vi "Find Yellow.vi"(6 "error in":errorcluster, 9 "SS File Path":path=path "C:/PokerSS/SS.png") -> (0 "error out":errorcluster, 3 "Yellow Player":dbl)   [LabVIEW 2015]
uses:
  <vilib>/vision/NI_Vision_Development_Module.lvlib
panel:
  in  "Grid for Yellow Player":dbl[][](array[numeric])=[[1041.0, 471.0, 1195.0, 510.0], [1226.0, 513.0, 1379.0, 553.0], [1368.0, 674.0, 1521.0, 715.0], [1235.0, 807.0, 1393.0, 856.0], [1004.0, 835.0, 1161.0, 885.0], [735.0, 844.0, 893.0, 885.0], [518.0, 810.0, 680.0, 854.0], [363.0, 668.0, 522.0, 709.0], [505.0, 510.0, 662.0, 554.0], [697.0, 475.0, 855.0, 514.0]]
  out "Found Yellow":bool
  in  "Minimum Match Score (Find Yellow)":sgl=800.0
  in  "Number of Matches Requested (Find Yellow)":i32=1
  in  "Search Strategy (Find Yellow)":u32(ring) items=["Conservative", "Balance", "Aggressive", "Very Aggressive"]
  in  "Color Sensitivity (Find Yellow)":u32(ring) items=["Low Sensitivity", "Medium Sensitivity", "High Sensitivity"]
  in  "File Path for Template":path=path "C:/Users/Bob Dabalina/Documents/Labview/Poker Hand2/YellowTemplate1.png"
  in  "ROI Descriptor (Find Yellow)":T1={"Global Rectangle"=[0, 0, 1919, 1079], "Contours"=[{"ID"=enum."External", "Type"=12, "Coordinates"=[0, 0, 1919, 1079, 0]}]} {"Contours"."Type" items=["No Selection", "Point", "Line", "Rectangle", "Oval", "Polygon", "Freehand Region", "Annulus", "Unused2", "Unused3", "Broken Line", "Freehand Line", "Rotated Rectangle"]}
  out "Image Out":T2(plugin-control)
  out "Matches (Find Yellow)":T3(array[cluster]) {"Bounding Box"."y" format="%.2f"; "Bounding Box"."x" format="%.2f"; "Position"."y" format="%.2f"; "Position"."x" format="%.2f"; "Score" format="%.2f"; "Scale" format="%.2f"; "Angle" format="%.2f"}
  # "x,y,x,y"
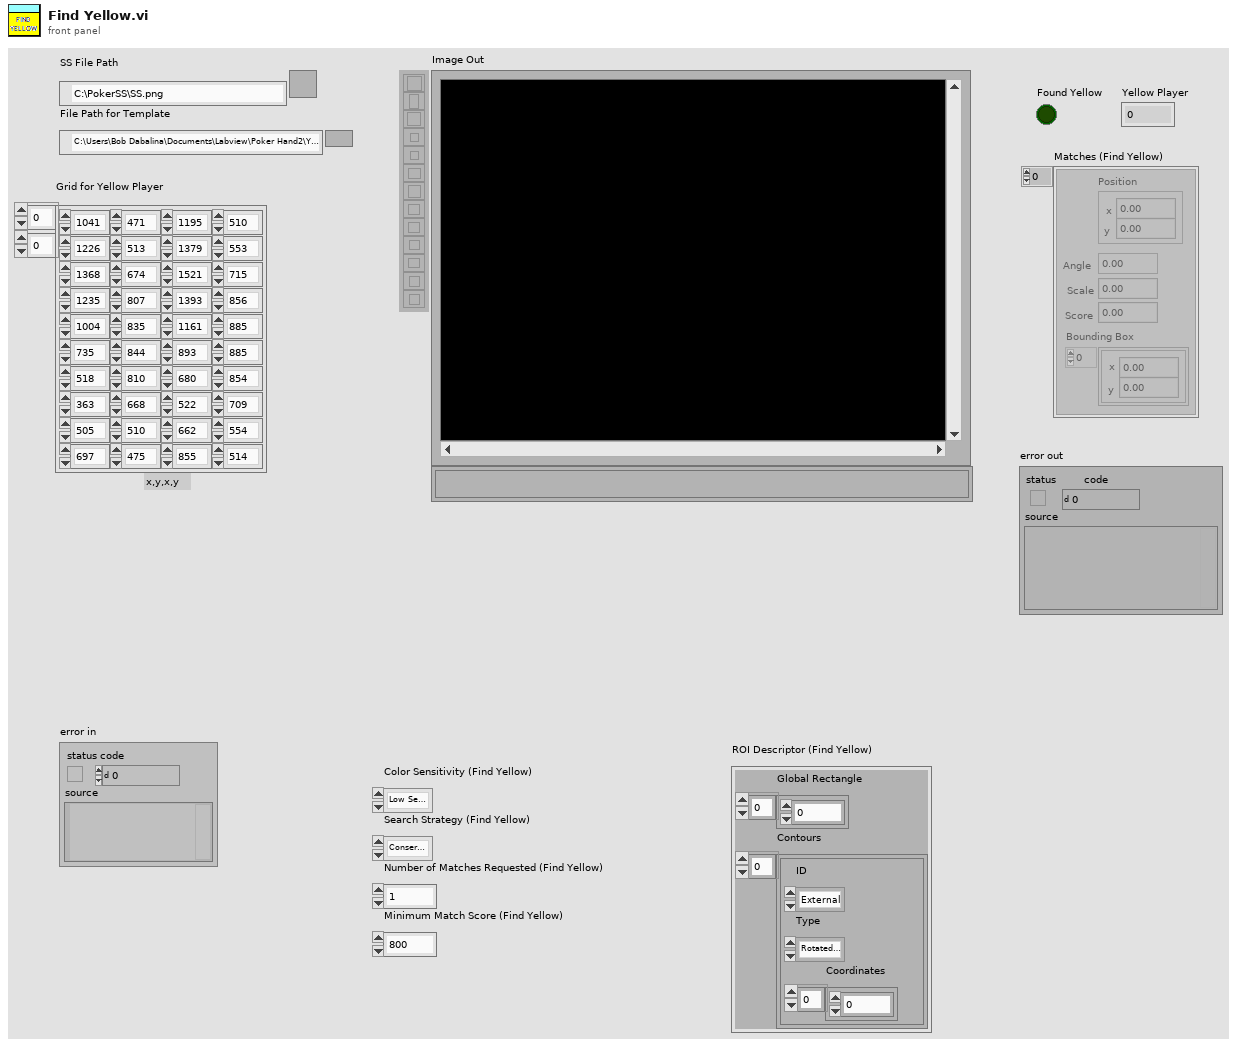
[diagram p1: front panel]
types:
  T1 = cluster{"Global Rectangle":i32[], "Contours":cluster{"ID":enum32{"External", "Internal"}, "Type":u32, "Coordinates":i32[]}[]}
  T2 = typedef "IMAQ Image.ctl" = refnum<image>
  T3 = cluster{"Position":cluster{"x":sgl, "y":sgl}, "Angle":sgl, "Scale":sgl, "Score":sgl, "Bounding Box":cluster{"x":sgl, "y":sgl}[]}[]
  T4 = typedef "Image Type" = u32
  T5 = cluster{"Position":cluster{"x":sgl, "y":sgl}, "Angle":sgl, "Scale":sgl, "Score":sgl, "Bounding Box":cluster{"x":sgl, "y":sgl}[]}
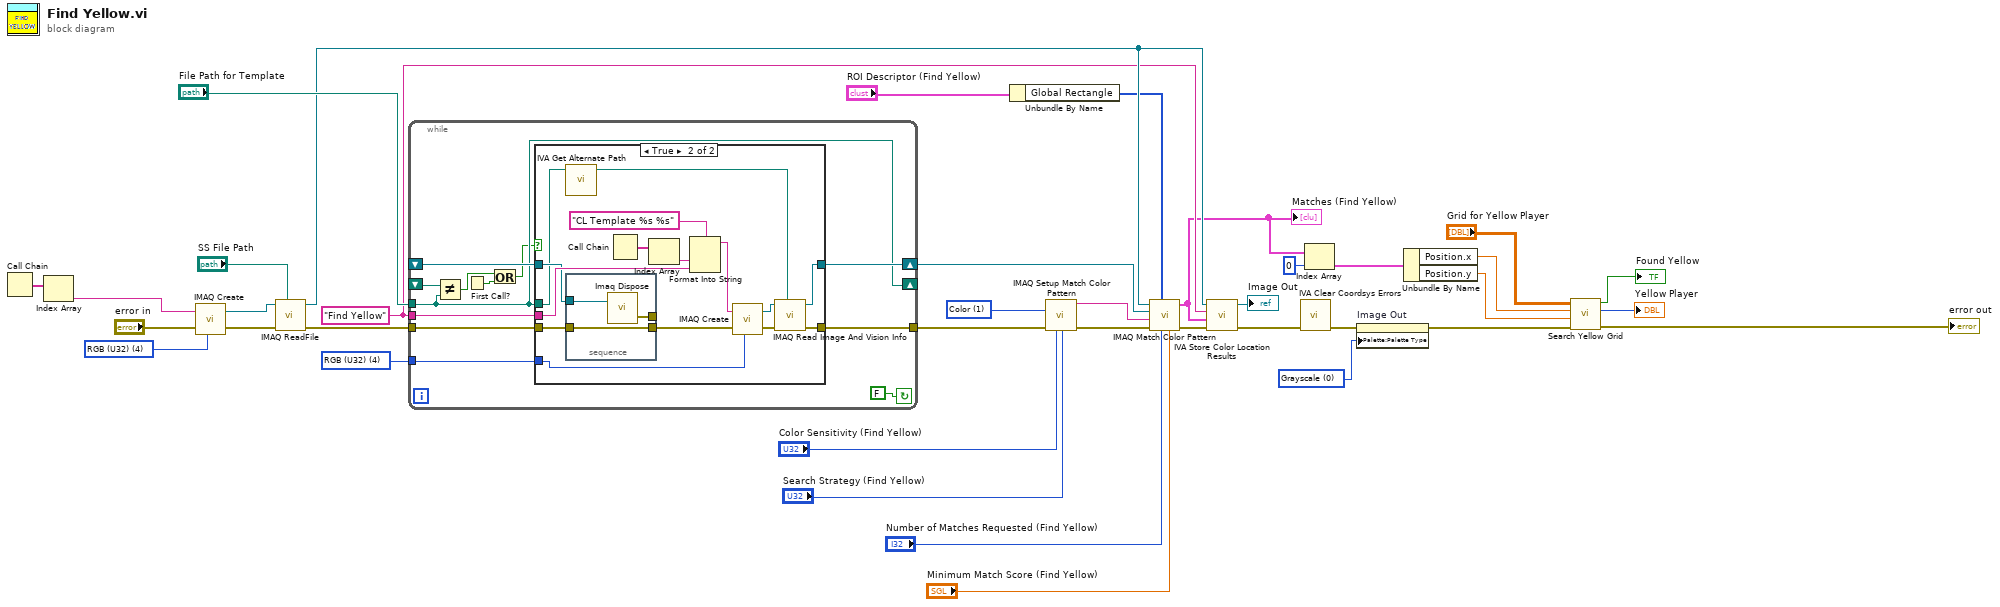
[diagram p0: block diagram]
diagram:
  w12 = u32 0 items=["Grayscale", "Binary", "Gradient", "Rainbow", "Temperature", "User Defined", "Binary 16 Bit", "Gradient 16 Bit", "Rainbow 16 Bit", "Temperature 16 Bit", "User Defined 16 Bit"] ("Palette Type")
  w21 = "Find Yellow" ("Step Name")
  w25 = T4 4 items=["Grayscale (U8)", "Grayscale (I16)", "Grayscale (SGL)", "Complex (CSG)", "RGB (U32)", "HSL (U32)", "RGB (U64)"] ("Image Type")
  w29 = u32 1 items=["Color and Shape", "Color", "Shape"] ("Match Feature Mode")
  w32 = T4 4 items=["Grayscale (U8)", "Grayscale (I16)", "Grayscale (SGL)", "Complex (CSG)", "RGB (U32)", "HSL (U32)", "RGB (U64)", "Grayscale (U16)"] ("Image Type")
  n1 = Call Chain() -> (call chain=w34:string[])
  n2 = Index Array(array=w34) -> (element=w33:string)  [unwired: 1 in]
  n3 = call "IMAQ Create"("Image Name"=w33, "Image Type"=w32, "error in (no error)"="error in") -> ("New Image"=w37:T2, "error out"=w36:errorcluster)  [unwired: 1 in, 1 out]
  n4 = call "IMAQ ReadFile"("File Path"="SS File Path", "error in (no error)"=w36, "Image"=w37) -> ("error out"=w38:errorcluster, "Image Out"=w22:T2)  [unwired: 2 in, 5 out]
  n5 = while {
    shift-right: [w50] -> w17
    shift-left: _ -> [w49]
    tunnel: [w47] -> w16
    tunnel: w38 -> [w46]
    tunnel: "File Path for Template" -> [w42]
    tunnel: w25 -> [w45]
    tunnel: w21 -> [w44]
    shift-right: [w42] -> _
    shift-left: _ -> [w43]
    stop <- FALSE continue-if-true
    n6 = Not Equal?(x=w43, y=w42) -> (x != y?=w40:bool)
    n7 = First Call?() -> (First Call?: T/F=w41:bool)
    n8 = Or(x=w40, y=w41) -> (x .or. y?=w39:bool)
    n9 = case shown="True" w39 {
      tunnel: [w52 w65] -> w50
      tunnel: w49 -> [w52 w57]
      tunnel: [w51 w62] -> w47
      tunnel: w46 -> [w51 w56]
      tunnel: w45 -> [_ w61]
      tunnel: w44 -> [_ w58]
      tunnel: w42 -> [_ w54]
      frame False {
      }
      frame True {
        n10 = call <vilib>:"IVA Get Alternate Path.vi"("Path In"=w54) -> ("Path Out"=w53:path)  [unwired: 10 out]
        n11 = stacked-sequence {
          tunnel: w57 -> [w70]
          tunnel: w56 -> [w69]
          tunnel: [w69] -> w55
          tunnel: [w68] -> _
          frame #0 {
            n12 = call "Imaq Dispose"("Image"=w70) -> ("error out"=w68:errorcluster)  [unwired: 2 in, 3 out]
          }
        }
        n13 = Call Chain() -> (call chain=w60:string[])
        n14 = Index Array(array=w60) -> (element=w59:string)  [unwired: 1 in]
        n15 = Format Into String(format string="CL Template %s %s" ("Image Name"), w59, w58) -> (resulting string=w67:string)  [unwired: 2 in, 1 out]
        n16 = call "IMAQ Create"("Image Name"=w67, "Image Type"=w61, "error in (no error)"=w55) -> ("New Image"=w64:T2, "error out"=w63:errorcluster)  [unwired: 1 in, 1 out]
        n17 = call "IMAQ Read Image And Vision Info"("File Path"=w53, "error in (no error)"=w63, "Image"=w64) -> ("error out"=w62:errorcluster, "Image Out"=w65:T2)  [unwired: 1 in, 6 out]
      }
    }
  }
  n18 = Unbundle By Name("ROI Descriptor (Find Yellow)") -> ("Global Rectangle"=w18:i32[])
  n19 = call "IMAQ Setup Match Color Pattern"("Match Feature Mode"=w29, "error in (no error)"=w16, "Color Sensitivity"="Color Sensitivity (Find Yellow)", "Search Strategy"="Search Strategy (Find Yellow)") -> ("Match Color Pattern Setup Data"=w20:string, "error out"=w19:errorcluster)  [unwired: 5 in, 5 out]
  n20 = call "IMAQ Match Color Pattern"("Minimum Match Score"="Minimum Match Score (Find Yellow)", "Number of Matches Requested"="Number of Matches Requested (Find Yellow)", "Optional Rectangle"=w18, "error in (no error)"=w19, "Match Color Pattern Setup Data"=w20, "Template Image"=w17, "Image"=w22) -> ("error out"=w23:errorcluster, "Matches"=w10:T3)  [unwired: 3 out]
  "Matches (Find Yellow)" <- w10
  n21 = call <vilib>:"IVA Store Color Location Results.vi"("error in (no error)"=w23, "Matches"=w10, "Step Name"=w21, "Image in"=w22) -> ("error out"=w15:errorcluster, "Image dup"=→"Image Out":T2)  [unwired: 6 out]
  n22 = call <vilib>:"IVA Clear Coordsys Errors.vi"("error in (no error)"=w15) -> ("error out"=w14:errorcluster)  [unwired: 10 in]
  n23 = Index Array(array=w10, index=0) -> (element=w8:T5)
  n24 = property on="Image Out" class="ImageControl"(error in=w14, "Palette:Palette Type"=w12) -> (error out=w7:errorcluster)  [unwired: 1 in, 1 out]
  n25 = Unbundle By Name(w8) -> ("Position.x"=w4:sgl, "Position.y"=w3:sgl)
  n26 = call "Search Yellow Grid.vi"("error in (no error)"=w7, "y"=w3, "x"=w4, "Grid for Yellow Player"="Grid for Yellow Player") -> ("error out"=→"error out":errorcluster, "Yellow Player #"=→"Yellow Player":i32, "Found in Grid"=→"Found Yellow":bool)  [unwired: 5 in]
